vi "SetMeasRange.vi"(2 "Channel Setting 1":T1 {"Meas Range" items=["-0.1 V~+0.1 V"=0.1, "-0.2 V~0.2 V"=0.2, "-0.5 V~+0.5 V"=0.5, "-1 V~+1 V"=1.0, "-2 V~+2 V"=2.0, "-5 V~+5 V"=5.0, "-10 V~+10 V"=10.0]; "Vertical\nPosition (Div)" min=-5.0 max=5.0 step=0.01 scale=-5.0..5.0 scale format="%.2f"; "Scale\n  Volts/Div" scale=0.01..20.0}, 3 "Error In":errorcluster caption="错误输入", 4 "Task In":refnum<k21> caption="任务输入", 5 "Channel Setting 0":T1 {"Meas Range" items=["-0.1 V~+0.1 V"=0.1, "-0.2 V~0.2 V"=0.2, "-0.5 V~+0.5 V"=0.5, "-1 V~+1 V"=1.0, "-2 V~+2 V"=2.0, "-5 V~+5 V"=5.0, "-10 V~+10 V"=10.0]; "Vertical\nPosition (Div)" min=-5.0 max=5.0 step=0.01 scale=-5.0..5.0 scale format="%.2f"; "Scale\n  Volts/Div" scale=0.01..20.0}) -> (0 "Error Out":errorcluster caption="错误输出", 1 "Task Out":refnum<k21> caption="任务输出")   [LabVIEW 2012]
uses:
  <resource>/objmgr/daqmx.rc
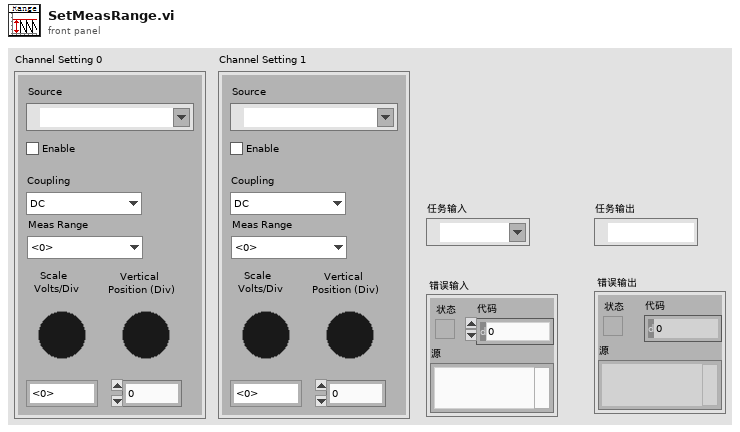
[diagram p1: front panel]
types:
  T1 = cluster{"physical channels":tag, "Enable":bool, "Coupling":enum16{"DC", "AC"}, "    Scale\n  Volts/Div  ":dbl, "    Vertical\nPosition (Div)":dbl, "Meas Range":dbl}
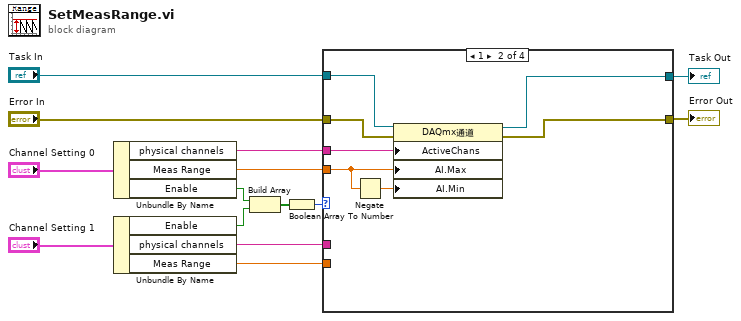
[diagram p0: block diagram]
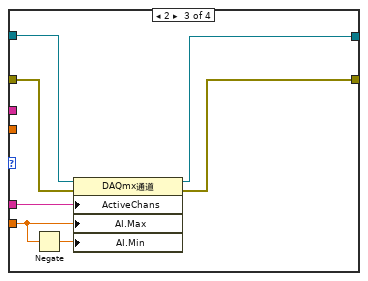
[diagram p3: hidden frame]
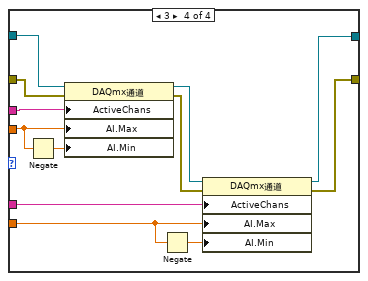
[diagram p4: hidden frame]
diagram:
  n1 = Unbundle By Name("Channel Setting 0") -> ("physical channels"=w7:tag, "Meas Range"=w6:dbl, "Enable"=w3:bool)
  n2 = Unbundle By Name("Channel Setting 1") -> ("Enable"=w2:bool, "physical channels"=w11:tag, "Meas Range"=w5:dbl)
  n3 = Build Array(w3, w2) -> (w4:bool[])
  n4 = Boolean Array To Number(Boolean array=w4) -> (number=w1:u32)
  n5 = case shown="1" w1 {
    tunnel: w7 -> [_ w21 _ w41]
    tunnel: w11 -> [_ _ w27 w35]
    tunnel: [w15 w18 w25 w32] -> w14
    tunnel: [w16 w17 w24 w31] -> w10
    tunnel: "Error In" -> [w16 w22 w28 w39]
    tunnel: "Task In" -> [w15 w23 w29 w38]
    tunnel: w6 -> [_ w20 _ w40]
    tunnel: w5 -> [_ _ w26 w33]
    frame 0, Default {
    }
    frame 1 {
      n6 = Negate(x=w20) -> (-x=w19:dbl)
      n7 = property class="DAQmx通道"(reference=w23, error in=w22, "ActiveChans"=w21, "AI.Max"=w20, "AI.Min"=w19) -> (reference out=w18:refnum<k21>, error out=w17:errorcluster)
    }
    frame 2 {
      n8 = Negate(x=w26) -> (-x=w30:dbl)
      n9 = property class="DAQmx通道"(reference=w29, error in=w28, "ActiveChans"=w27, "AI.Max"=w26, "AI.Min"=w30) -> (reference out=w25:refnum<k21>, error out=w24:errorcluster)
    }
    frame 3 {
      n10 = Negate(x=w40) -> (-x=w42:dbl)
      n11 = property class="DAQmx通道"(reference=w38, error in=w39, "ActiveChans"=w41, "AI.Max"=w40, "AI.Min"=w42) -> (reference out=w37:refnum<k21>, error out=w36:errorcluster)
      n12 = Negate(x=w33) -> (-x=w34:dbl)
      n13 = property class="DAQmx通道"(reference=w37, error in=w36, "ActiveChans"=w35, "AI.Max"=w33, "AI.Min"=w34) -> (reference out=w32:refnum<k21>, error out=w31:errorcluster)
    }
  }
  "Task Out" <- w14
  "Error Out" <- w10
